vi "FindNameInTree.vi"() -> ()   [LabVIEW 2013]
doc: "Provides a mechanism to allow the user to specify a string to be searched for. Tree items containing a match are highlighted. Also, a count of matching tree items is displayed, along with a count of all tree items."
uses:
  <vilib>/Utility/miscctls.llb/LVSelectionTypeDef.ctl
  FindName Task_Manager.lvlib
panel:
  out "Found/Total =":string
  in  "Data Tree":refnum<vi>
  in  "NameToFind":string caption="Find ="
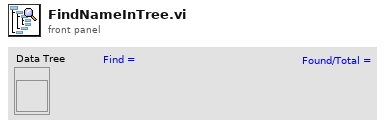
[diagram p1: front panel]
types:
  T1 = typedef "LVSelectionTypeDef.ctl" = cluster{"Selection Start":u32, "Selection End":u32}
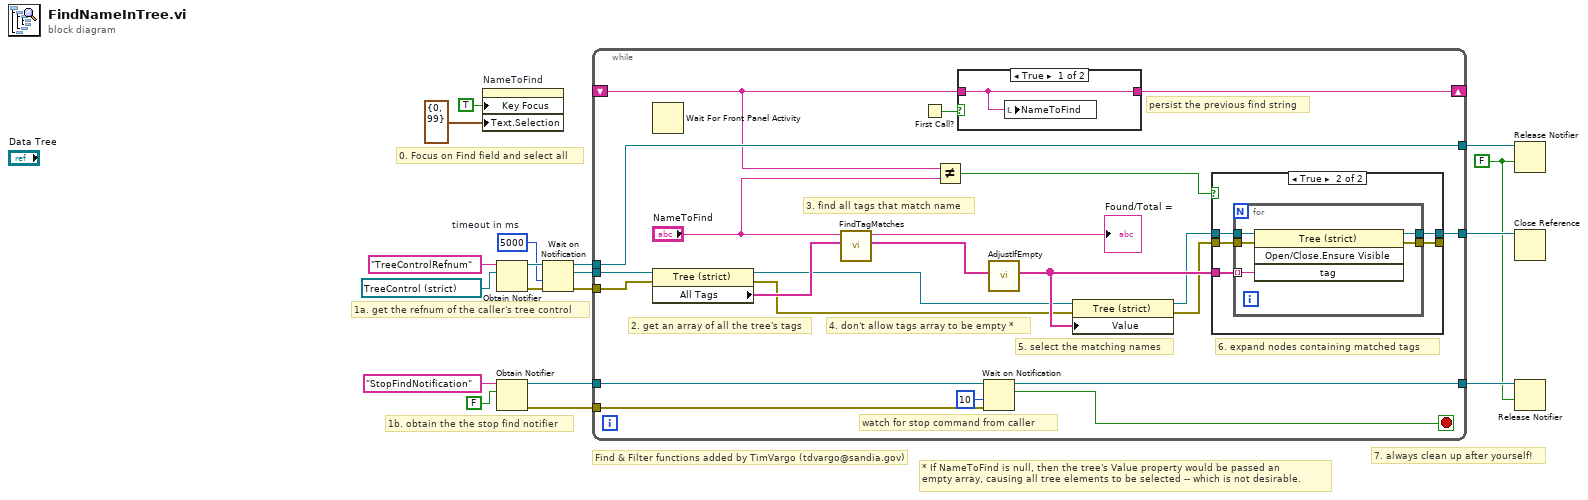
[diagram p0: block diagram]
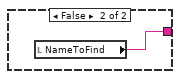
[diagram p3: hidden frame]
diagram:
  w1 = FALSE ("force destroy? (F)")
  w5 = 5000  # timeout in ms
  # "Find & Filter functions added by TimVargo (tdvargo@sandia.gov)"
  # "* If NameToFind is null, then the tree's Value property would be passed an \nempty array, causing all tree elements to be selected -- which is not desirable."
  # "1b. obtain the the stop find notifier"
  # "0. Focus on Find field and select all"
  # "7. always clean up after yourself!"
  # "1a. get the refnum of the caller's tree control"
  n1 = property on="NameToFind" class="Str"("Key Focus"=TRUE, "Text.Selection"=T1 {"Selection Start"=0, "Selection End"=99}) -> ()  [unwired: 2 in, 2 out]
  n2 = Obtain Notifier(name (unnamed)="TreeControlRefnum", notification data type=refnum<vi> refnum ("Data Tree")) -> (notifier out=w15:refnum<notifier>, error out=w16:errorcluster)  [unwired: 2 in, 1 out]
  n3 = Obtain Notifier(name (unnamed)="StopFindNotification", notification data type=FALSE) -> (notifier out=w4:refnum<notifier>, error out=w3:errorcluster)  [unwired: 2 in, 1 out]
  n4 = Wait on Notification(notifier=w15, timeout in ms (-1)=w5, error in (no error)=w16) -> (notifier out=w13:refnum<notifier>, notification=w14:refnum<vi>, error out=w10:errorcluster)  [unwired: 1 in, 1 out]
  n5 = while {
    tunnel: w14 -> [w39]
    tunnel: w13 -> [w38]
    tunnel: [w38] -> w12
    tunnel: [w23] -> w11
    tunnel: w10 -> [w19]
    shift-right: [w35] -> _
    shift-left: _ -> [w20]
    tunnel: w4 -> [w33]
    tunnel: w3 -> [w32]
    tunnel: [w31] -> w2
    stop <- w28 stop-if-true
    # "6. expand nodes containing matched tags"
    # "4. don't allow tags array to be empty *"
    # "watch for stop command from caller"
    # "persist the previous find string"
    # "3. find all tags that match name"
    # "5. select the matching names"
    # "2. get an array of all the tree's tags"
    n6 = Wait For Front Panel Activity() -> ()  [unwired: 3 in, 1 out]
    n7 = property class="Tree (strict)"(reference=w39, error in=w19) -> (reference out=w21:refnum<vi>, error out=w22:errorcluster, "All Tags"=w34:string[])
    n8 = call "FindTagMatches.vi"("All Tags"=w34, "NameToFind"="NameToFind") -> ("Found"=w37:string[], "ResultString"=→"Found/Total =":string)  [unwired: 7 in, 1 out]
    n9 = First Call?() -> (First Call?: T/F=w36:bool)
    n10 = Not Equal?(x=w20, y="NameToFind") -> (x != y?=w26:bool)
    n11 = case shown="True" w36 {
      tunnel: [w53 w54] -> w35
      tunnel: w20 -> [w53 _]
      frame True {
        n12 = local write "NameToFind"(w53) -> ()
      }
      frame False {
        n13 = local read "NameToFind"() -> (w54:string)
      }
    }
    n14 = Wait on Notification(notifier=w33, timeout in ms (-1)=10, error in (no error)=w32) -> (notifier out=w31:refnum<notifier>, notification=w28:bool)  [unwired: 1 in, 2 out]
    n15 = call "AdjustIfEmpty.vi"("Found"=w37) -> ("FoundAdj"=w29:string[])  [unwired: 10 in]
    n16 = property class="Tree (strict)"(reference=w21, error in=w22, "Value"=w29) -> (reference out=w25:refnum<vi>, error out=w24:errorcluster)
    n17 = case shown="True" w26 {
      tunnel: [w41 w47] -> _
      tunnel: w24 -> [w41 w46]
      tunnel: w25 -> [w42 w45]
      tunnel: [w42 w44] -> w23
      tunnel: w29 -> [_ w43]
      frame False {
      }
      frame True {
        n18 = for {
          tunnel: [w52] -> w47
          tunnel: w46 -> [w51]
          tunnel: w45 -> [w50]
          tunnel: [w49] -> w44
          tunnel: w43 -> [w48] mode=indexing
          n19 = invoke class="Tree (strict)" method="Open/Close.Ensure Visible"(reference=w50, error in=w51, "tag"=w48) -> (reference out=w49:refnum<vi>, error out=w52:errorcluster)  [unwired: 1 in, 2 out]
        }
      }
    }
  }
  n20 = Release Notifier(notifier=w12, force destroy? (F)=w1) -> ()  [unwired: 1 in, 3 out]
  n21 = Close Reference(reference=w11) -> ()  [unwired: 1 in, 1 out]
  n22 = Release Notifier(notifier=w2, force destroy? (F)=w1) -> ()  [unwired: 1 in, 3 out]
